vi "Get Dir.vi"(11 "ConfigJSON in":refnum<class "ConfigJSON.lvclass">) -> (2 "Config Dir":path, 3 "ConfigJSON out":refnum<class "ConfigJSON.lvclass">)   [LabVIEW 2019, in "ConfigJSON.lvclass"]
uses:
  ConfigJSON.lvclass
  ConfigJSON.lvclass/ConfigJSON.ctl
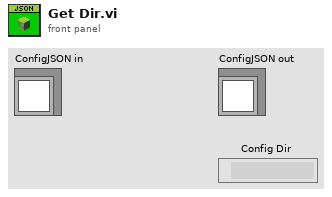
[diagram p1: front panel]
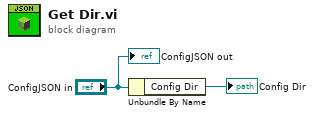
[diagram p0: block diagram]
diagram:
  n1 = Unbundle By Name("ConfigJSON in") -> ("Config Dir"=→"Config Dir":path)
  "ConfigJSON out" <- "ConfigJSON in"
